vi "Extract Debug Client Data.vi"(11 "AppMgr in":refnum<class "Application Manager.lvclass">) -> (2 "IP Address":string, 3 "DC_UID":T1)   [LabVIEW 2017, in "Application Manager.lvclass"]
doc: "Extract the Debug Client UID and the IP Address from the Debug Client data"
uses:
  Application Manager.lvclass
  Common VIs/DC_UID.ctl
  C:/Program Files (x86)/National Instruments/LabVIEW 2017/vi.lib/addons/_Workers/Library/Classes/Worker/Worker.lvclass
  <vilib>/addons/_Workers/Library/Classes/Worker/Worker.lvclass/Worker.ctl
  <vilib>/addons/_Workers/Library/Classes/Message/Message.lvclass/Message.ctl
  <vilib>/addons/_Workers/Library/Classes/Worker/Worker.lvclass
  <vilib>/addons/_Workers/Library/Classes/Message/Message.lvclass
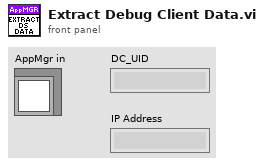
[diagram p1: front panel]
types:
  T1 = typedef "DC_UID.ctl" = string
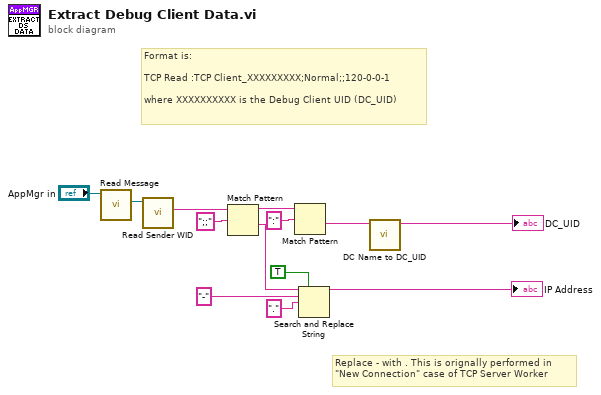
[diagram p0: block diagram]
diagram:
  # "Replace - with . This is orignally performed in \n\"New Connection\" case of TCP Server Worker"
  # "Format is:\n\nTCP Read :TCP Client_XXXXXXXXX;Normal;;120-0-0-1\n\nwhere XXXXXXXXXX is the Debug Client UID (DC_UID)"
  n1 = call <vilib>:"Read Message.vi"("Worker"="AppMgr in") -> ("Message"=w8:refnum<class "Message.lvclass">)  [unwired: 9 in, 1 out]
  n2 = call <vilib>:"Read Sender WID.vi"("Message"=w8) -> ("Sender WID"=w7:string)  [unwired: 9 in, 1 out]
  n3 = Match Pattern(string=w7, regular expression=";;") -> (before substring=w4:string, after substring=w12:string)  [unwired: 1 in, 2 out]
  n4 = Match Pattern(string=w4, regular expression=":") -> (after substring=w2:string)  [unwired: 1 in, 3 out]
  n5 = Search and Replace String(replace all?=TRUE ("replace all? (F)"), input string=w12, search string="-", replace string="." ("replace string (\"\")")) -> (result string=→"IP Address":string)  [unwired: 4 in, 3 out]
  n6 = call "DC Name to DC_UID.vi"("DC Name"=w2) -> ("DC_UID"=→"DC_UID":T1)  [unwired: 10 in]
